vi "SetAlarmsSettings.vi"(7 "TYPE":T2, 10 "SettinganalogComp":T1, 11 "Sig_AI in":refnum<class "AI.lvclass">) -> (3 "Sig_AI out":refnum<class "AI.lvclass">)   [LabVIEW 2019, in "AI.lvclass"]
uses:
  AI.lvclass
  AI Alarm Type.ctl
  TypeDef/ConfigAnalogComp.ctl
  AI.lvclass/AI.ctl
  AnalogComparator_class/AnalogComparator.lvclass/AnalogComparator.ctl
  AnalogComparator_class/AnalogComparator.lvclass
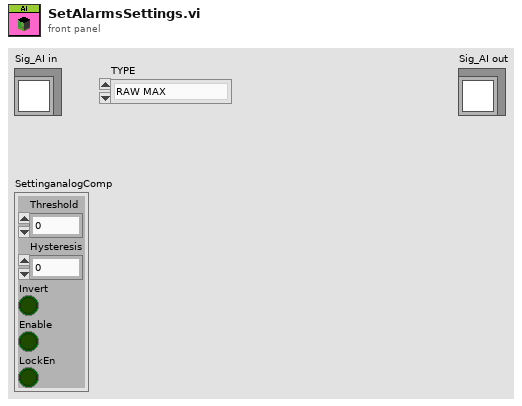
[diagram p1: front panel]
types:
  T1 = typedef "ConfigAnalogComp.ctl" = cluster{"Threshold":dbl, "Hysteresis":dbl, "Invert":bool, "Enable":bool, "LockEn":bool}
  T2 = typedef "AnalogComparator.lvclass/AI Alarm Type.ctl" = enum16{"RAW MAX", "RAW MIN", "HIHI", "HI", "LO", "LOLO"}
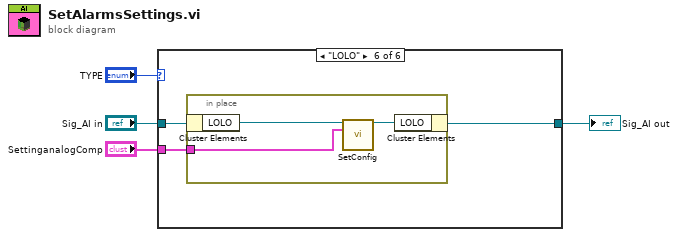
[diagram p0: block diagram]
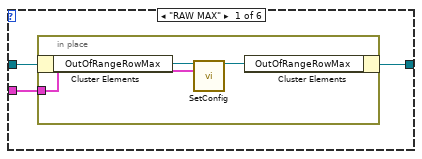
[diagram p2: hidden frame]
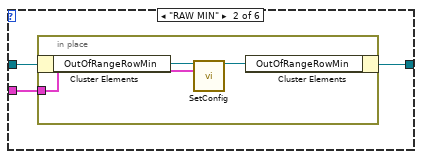
[diagram p3: hidden frame]
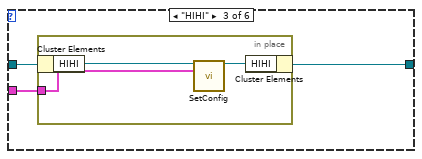
[diagram p4: hidden frame]
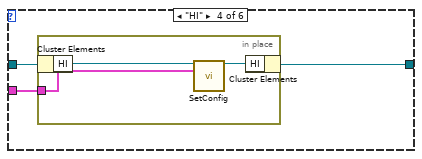
[diagram p5: hidden frame]
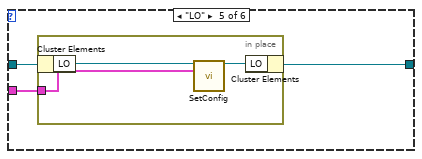
[diagram p6: hidden frame]
diagram:
  n1 = case shown="\"LOLO\"" "TYPE" {
    tunnel: "Sig_AI in" -> [w7 w13 w19 w25 w31 w37]
    tunnel: [w6 w12 w18 w24 w30 w36] -> w3
    tunnel: "SettinganalogComp" -> [w5 w11 w17 w23 w29 w35]
    frame "RAW MAX" {
      n2 = in-place {
        in-place-border: w5 -> [w8]
        n3 = in-place-cluster #1(w7) -> ("OutOfRangeRowMax"=w10:refnum<class "AnalogComparator.lvclass">)
        n4 = call "SetConfig.vi"("class data in"=w10, "SettinganalogComp"=w8) -> ("class data out"=w9:refnum<class "AnalogComparator.lvclass">)  [unwired: 13 in]
        n5 = in-place-cluster #1("OutOfRangeRowMax"=w9) -> (w6:refnum<class "AI.lvclass">)
      }
    }
    frame "RAW MIN" {
      n6 = in-place {
        in-place-border: w11 -> [w14]
        n7 = in-place-cluster #2(w13) -> ("OutOfRangeRowMin"=w16:refnum<class "AnalogComparator.lvclass">)
        n8 = call "SetConfig.vi"("class data in"=w16, "SettinganalogComp"=w14) -> ("class data out"=w15:refnum<class "AnalogComparator.lvclass">)  [unwired: 13 in]
        n9 = in-place-cluster #2("OutOfRangeRowMin"=w15) -> (w12:refnum<class "AI.lvclass">)
      }
    }
    frame "HIHI" {
      n10 = in-place {
        in-place-border: w17 -> [w20]
        n11 = in-place-cluster #3(w19) -> ("HIHI"=w22:refnum<class "AnalogComparator.lvclass">)
        n12 = call "SetConfig.vi"("class data in"=w22, "SettinganalogComp"=w20) -> ("class data out"=w21:refnum<class "AnalogComparator.lvclass">)  [unwired: 13 in]
        n13 = in-place-cluster #3("HIHI"=w21) -> (w18:refnum<class "AI.lvclass">)
      }
    }
    frame "HI" {
      n14 = in-place {
        in-place-border: w23 -> [w26]
        n15 = in-place-cluster #4(w25) -> ("HI"=w28:refnum<class "AnalogComparator.lvclass">)
        n16 = call "SetConfig.vi"("class data in"=w28, "SettinganalogComp"=w26) -> ("class data out"=w27:refnum<class "AnalogComparator.lvclass">)  [unwired: 13 in]
        n17 = in-place-cluster #4("HI"=w27) -> (w24:refnum<class "AI.lvclass">)
      }
    }
    frame "LO" {
      n18 = in-place {
        in-place-border: w29 -> [w32]
        n19 = in-place-cluster #5(w31) -> ("LO"=w34:refnum<class "AnalogComparator.lvclass">)
        n20 = call "SetConfig.vi"("class data in"=w34, "SettinganalogComp"=w32) -> ("class data out"=w33:refnum<class "AnalogComparator.lvclass">)  [unwired: 13 in]
        n21 = in-place-cluster #5("LO"=w33) -> (w30:refnum<class "AI.lvclass">)
      }
    }
    frame "LOLO" {
      n22 = in-place {
        in-place-border: w35 -> [w38]
        n23 = in-place-cluster #6(w37) -> ("LOLO"=w40:refnum<class "AnalogComparator.lvclass">)
        n24 = call "SetConfig.vi"("class data in"=w40, "SettinganalogComp"=w38) -> ("class data out"=w39:refnum<class "AnalogComparator.lvclass">)  [unwired: 13 in]
        n25 = in-place-cluster #6("LOLO"=w39) -> (w36:refnum<class "AI.lvclass">)
      }
    }
  }
  "Sig_AI out" <- w3
